vi "Write FIB reheat log.vi"(4 "Capella HV Data Output":T1 {"Column Vac (Torr)" format="%.2e"; "Gun Vac (Torr)" format="%.2e"; "Lens2 Actual (V)" format="%.1f"; "Lens1 Actual (V)" format="%.1f"; "Emission Actual (uA)" format="%.3f"; "Extrator Actual (V)" format="%.1f"; "Tip Lifetime (uAhr)" format="%.2f"; "Lens2 Target (V)" format="%.1f"; "Lens1 Target (V)" format="%.1f"; "Faraday I (nA)" format="%.3f"; "Suppressor (V)" format="%.1f"; "Emission Target (uA)" format="%.3f"; "Extrator Target (V)" format="%.1f"; "Accelerator Actual (V)" format="%.1f"; "Accelerator Target (V)" format="%.1f"; "Filament (A)" format="%.2f"}, 6 "HV Data Output":T2 {"Tip Lifetime (hr)" format="%.2f"; "Lens2I (uA)" format="%.3f"; "Lens2 (V)" format="%.1f"; "Lens1I (uA)" format="%.3f"; "Lens1 (V)" format="%.1f"; "SuppI (uA)" format="%.3f"; "Suppressor (V)" format="%.1f"; "Emission (uA)" format="%.3f"; "Extrator (V)" format="%.1f"; "AccI (uA)" format="%.3f"; "Acclerator (V)" format="%.1f"; "Filament (A)" format="%.2f"}, 7 "Reheat Output":T3 {"Initial suppressor (V)" format="%.1f"; "Initial emission (uA)" format="%.3f"; "V/I Slope" format="%.2f"}, 8 "Reheat Parameters":T4={"Filament I (A)"=3.0, "Reheat time (s)"=45.0, "Emission (uA)"=2.2, "Calculate V/I slope"=TRUE, "Pre-calc delay (min)"=5.0, "Disable Reheat Retries"=FALSE, "Restore Voltages"=TRUE} {"Pre-calc delay (min)" format="%.2f"; "Emission (uA)" format="%.1f"; "Filament I (A)" format="%.2f"; "Reheat time (s)" format="%.1f"}, 9 "Reheat time":timestamp, 10 "Machine Type":u8(ring) items=["Feiss", "NVision", "Jeiss"], 11 "Log file path":path=path "C:/Program Files (x86)/FEI Company/BDS/LogHVData.log") -> ()   [LabVIEW 2018]
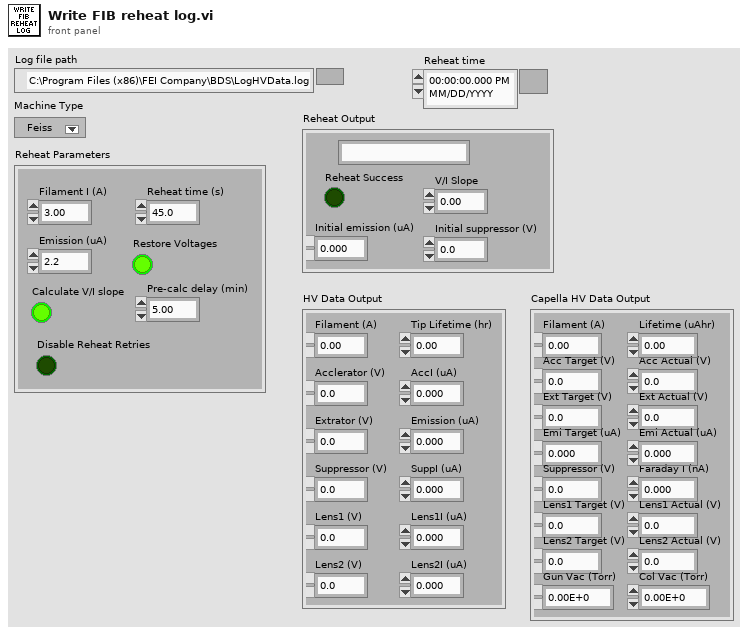
[diagram p1: front panel]
types:
  T1 = cluster{"Filament (A)":sgl, "Accelerator Target (V)":sgl, "Accelerator Actual (V)":sgl, "Extrator Target (V)":sgl, "Extrator Actual (V)":sgl, "Emission Target (uA)":sgl, "Emission Actual (uA)":sgl, "Suppressor (V)":sgl, "Faraday I (nA)":sgl, "Lens1 Target (V)":sgl, "Lens1 Actual (V)":sgl, "Lens2 Target (V)":sgl, "Lens2 Actual (V)":sgl, "Gun Vac (Torr)":sgl, "Column Vac (Torr)":sgl, "Tip Lifetime (uAhr)":sgl}
  T2 = cluster{"Filament (A)":sgl, "Acclerator (V)":sgl, "AccI (uA)":sgl, "Extrator (V)":sgl, "Emission (uA)":sgl, "Suppressor (V)":sgl, "SuppI (uA)":sgl, "Lens1 (V)":sgl, "Lens1I (uA)":sgl, "Lens2 (V)":sgl, "Lens2I (uA)":sgl, "Tip Lifetime (hr)":sgl}
  T3 = cluster{"Reheat finish time":string, "Reheat Success":bool, "Initial emission (uA)":sgl, "Initial suppressor (V)":sgl, "V/I Slope":sgl}
  T4 = cluster{"Filament I (A)":sgl, "Reheat time (s)":sgl, "Emission (uA)":sgl, "Calculate V/I slope":bool, "Pre-calc delay (min)":sgl, "Disable Reheat Retries":bool, "Restore Voltages":bool}
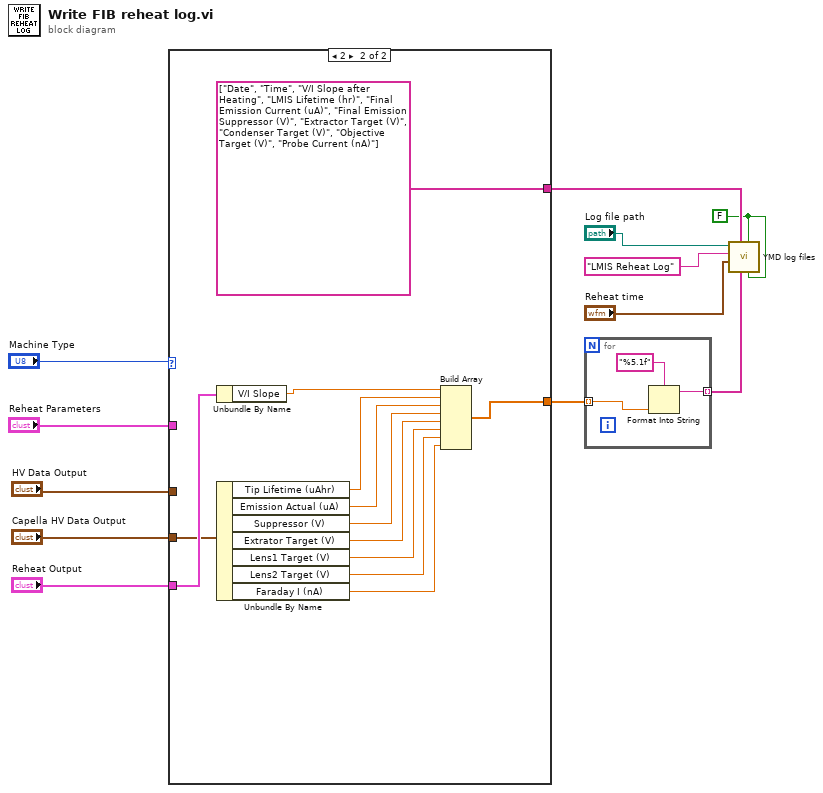
[diagram p0: block diagram]
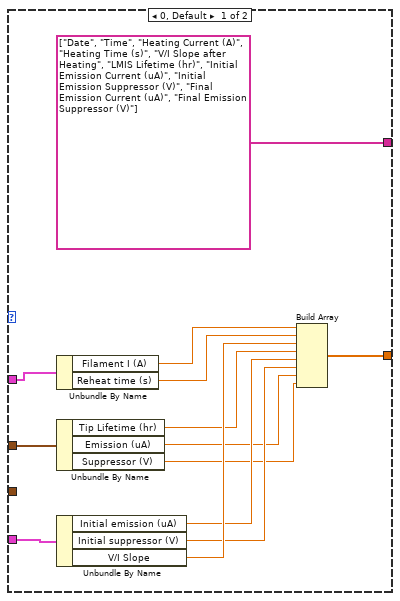
[diagram p2: hidden frame]
diagram:
  w1 = FALSE ("Month")
  n1 = case shown="2" "Machine Type" {
    tunnel: [string[] ["Date", "Time", "Heating Current (A)", "Heating Time (s)", "V/I Slope after Heating", "LMIS Lifetime (hr)", "Initial Emission Current (uA)", "Initial Emission Suppressor (V)", "Final Emission Current (uA)", "Final Emission Suppressor (V)"] string[] ["Date", "Time", "V/I Slope after Heating", "LMIS Lifetime (hr)", "Final Emission Current (uA)", "Final Emission Suppressor (V)", "Extractor Target (V)", "Condenser Target (V)", "Objective Target (V)", "Probe Current (nA)"]] -> w10
    tunnel: "Reheat Output" -> [w24 w36]
    tunnel: "Reheat Parameters" -> [w23 _]
    tunnel: [w17 w34] -> w6
    tunnel: "HV Data Output" -> [w16 _]
    tunnel: "Capella HV Data Output" -> [_ w30]
    frame 0, Default {
      n2 = Unbundle By Name(w23) -> ("Filament I (A)"=w22:sgl, "Reheat time (s)"=w21:sgl)
      n3 = Unbundle By Name(w16) -> ("Tip Lifetime (hr)"=w15:sgl, "Emission (uA)"=w14:sgl, "Suppressor (V)"=w13:sgl)
      n4 = Unbundle By Name(w24) -> ("Initial emission (uA)"=w19:sgl, "Initial suppressor (V)"=w18:sgl, "V/I Slope"=w20:sgl)
      n5 = Build Array(w22, w21, w20, w15, w19, w18, w14, w13) -> (w17:sgl[])
    }
    frame 2 {
      n6 = Unbundle By Name(w36) -> ("V/I Slope"=w35:sgl)
      n7 = Unbundle By Name(w30) -> ("Tip Lifetime (uAhr)"=w33:sgl, "Emission Actual (uA)"=w32:sgl, "Suppressor (V)"=w31:sgl, "Extrator Target (V)"=w29:sgl, "Lens1 Target (V)"=w28:sgl, "Lens2 Target (V)"=w27:sgl, "Faraday I (nA)"=w26:sgl)
      n8 = Build Array(w35, w33, w32, w31, w29, w28, w27, w26) -> (w34:sgl[])
    }
  }
  n9 = for {
    tunnel: w6 -> [w40] mode=indexing
    tunnel: [w39] -> w5 mode=indexing
    n10 = Format Into String(format string="%5.1f", w40) -> (resulting string=w39:string)  [unwired: 2 in, 1 out]
  }
  n11 = call "YMD log files.vi"("Day"=w1, "Month"=w1, "Input text array"=w5, "Input header array"=w10, "current time"="Reheat time", "Log file name"="LMIS Reheat Log", "Log file path"="Log file path") -> ()  [unwired: 5 in]
